vi "pH电极校准.vi"() -> ()   [LabVIEW 2016, in "斯坦道多参数.lvlib"]
uses:
  <vilib>/Utility/miscctls.llb/LVPointTypeDef.ctl
  <vilib>/Analysis/NI_AALBase.lvlib
panel:
  out "温度":dbl format="%#.2f"
  out "通讯状态":string
  out "电极状态标志":u16(ring) items=["OK", "第一点校正通过", "第二点校正通过", "校正失败,电极零点超出范围", "校正失败,电极斜率超出范围", "第三点校正通过"]
  in  "三点标液3":u16(ring)=6 caption="标液3" items=["TECH4.00", "TECH7.00", "TECH10.00", "NIST1.68", "NIST4.01", "NIST6.86", "NIST9.18", "NIST12.68"]
  in  "三点标液2":u16(ring)=5 caption="标液2" items=["TECH4.00", "TECH7.00", "TECH10.00", "NIST1.68", "NIST4.01", "NIST6.86", "NIST9.18", "NIST12.68"]
  in  "三点标液1":u16(ring)=4 caption="标液1" items=["TECH4.00", "TECH7.00", "TECH10.00", "NIST1.68", "NIST4.01", "NIST6.86", "NIST9.18", "NIST12.68"]
  out "第三点校准值":dbl
  in  "校准停止":bool
  in  "校准启动":bool
  out "第二点校准值":dbl
  out "第一点校准值":dbl
  out "提示":string
  in  "校准模式":enum16{"两点校准", "单点校准", "三点校准"}(ring)
  out "最小值":sgl format="%#.2f"
  out "最大值":sgl format="%#.2f"
  out "变异系数":dbl format="%#.6f"
  out "standard deviation":dbl caption="标准差" format="%#.2f"
  out "mean":dbl caption="均值" format="%#.2f"
  out "波形图表":sgl(graph) caption="历史曲线"
  out "当前检测值":dbl caption="测量值" format="%#.2f"
  out "标液2":dbl
  out "标液1":dbl
  out "当前信号值":dbl caption="信号值" format="%#.2f"
  out "偏移值补偿":dbl format="%#.2f"
  out "电极斜率":dbl format="%#.6f"
  out "电极零点":dbl format="%#.6f"
  # "酸碱度电极设定"
  # "℃"
  # "mV"
  # "mV"
  # "%"
  # "pH"
  # "请选择校准模式:"
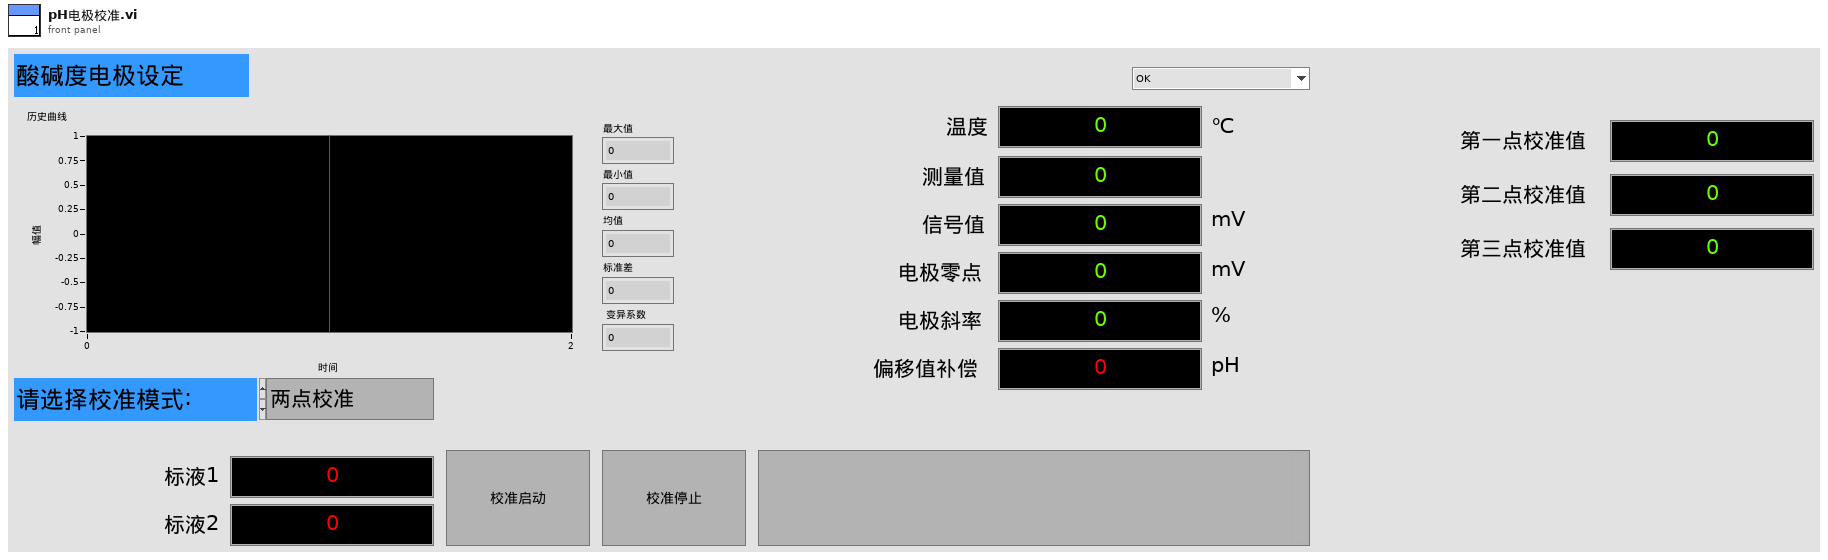
[diagram p1: front panel]
types:
  T1 = typedef "LVPointTypeDef.ctl" = cluster{"Horizontal":i16, "Vertical":i16}
  T2 = typedef "斯坦道多参数.lvlib/校准步骤.ctl" = enum16{"待机", "放置第一点标液", "第一点校准启动", "第一点校准写入", "第一点校准失败", "放置第二点标液", "第二点校准启动", "第二点校准写入", "第二点校准失败", "放置第三点标液", "第三点校准启动", "第三点校准写入", "第三点校准失败", "校准结果写入", "校准结束"}
  T3 = cluster{"电极状态标志":u16, "电极型号标志":u16, "酸碱度测量值":sgl, "温度测量值":sgl, "酸碱度信号值":sgl, "温度信号值":sgl, "酸碱度偏移修正值":sgl, "温度偏移修正值":sgl, "手动温度补偿值":sgl, "酸碱度电极零点":sgl, "酸碱度电极斜率":sgl, "第1点标准值记录":sgl, "第1点信号值记录":sgl, "第1点温度值记录":sgl, "第2点标准值记录":sgl, "第2点信号值记录":sgl, "第2点温度值记录":sgl, "命令滤波设定":u16, "温度模式":enum16{"ATC", "MTC"}, "生产批次":u16, "电极序号":u16, "串口地址":u16, "串口波特率":enum16{"9600", "19200", "115200"}, "串口校验位":enum16{"NONE", "ODD", "EVEN"}, "串口停止位":enum16{"1bit", "2bit"}, "第一点标准值":sgl, "第二点标准值":sgl}
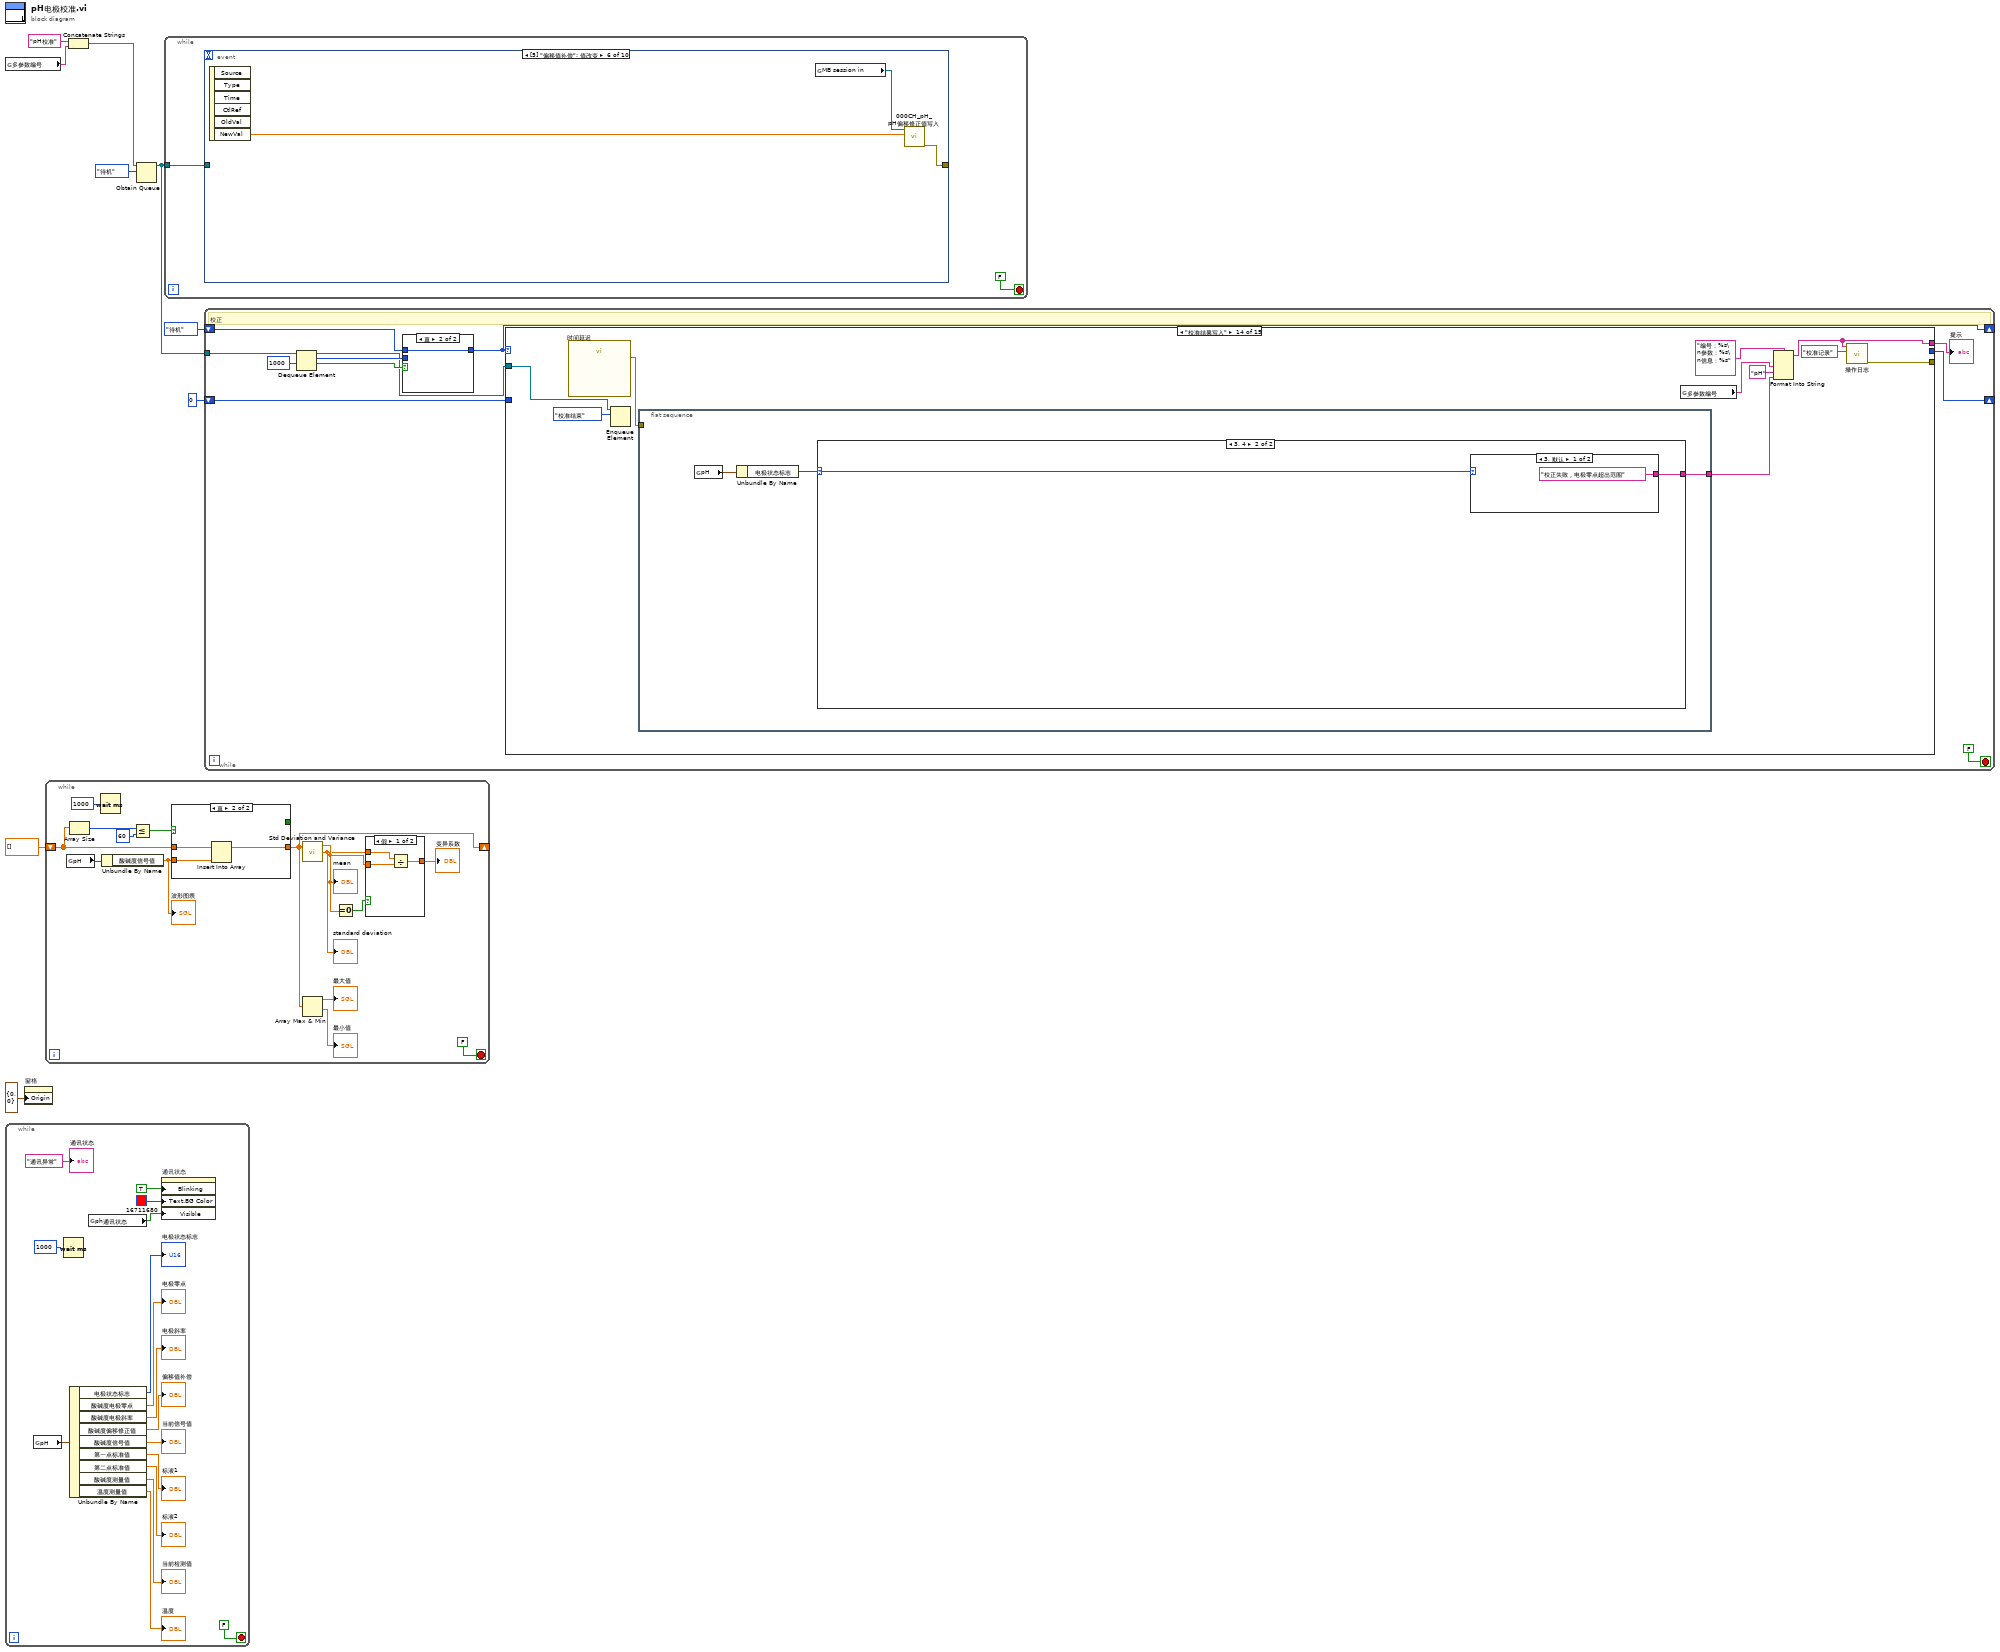
[diagram p0: block diagram]
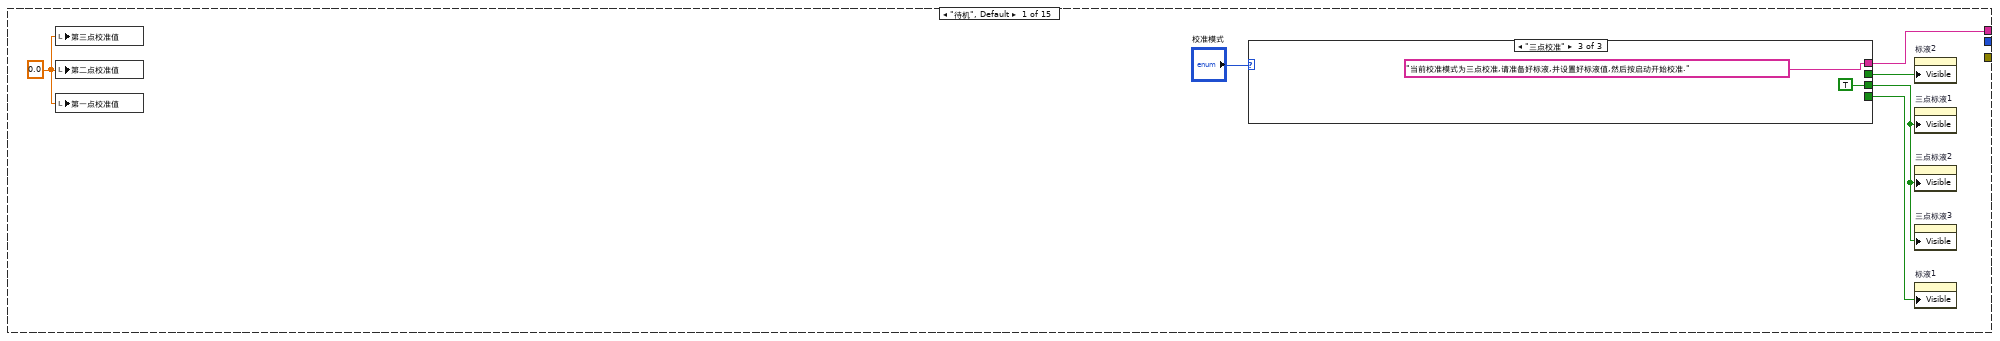
[diagram p3: hidden frame]
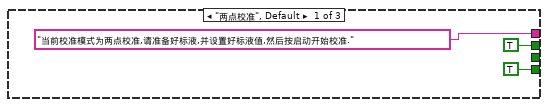
[diagram p4: hidden frame]
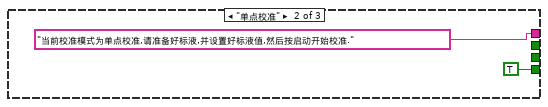
[diagram p5: hidden frame]
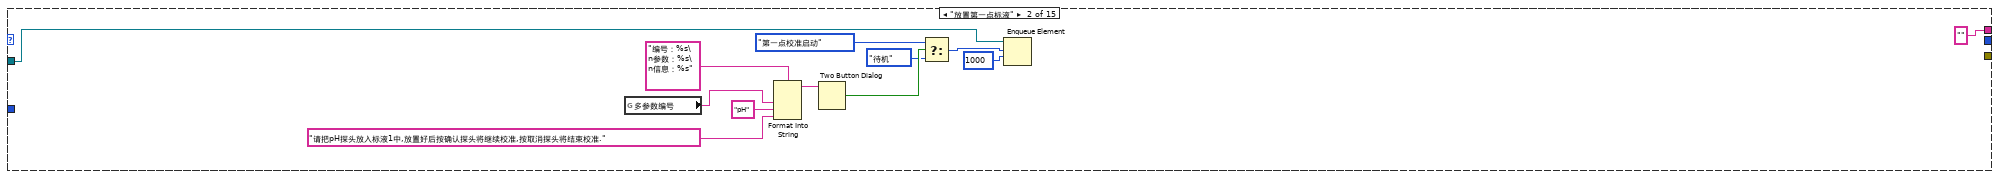
[diagram p6: hidden frame]
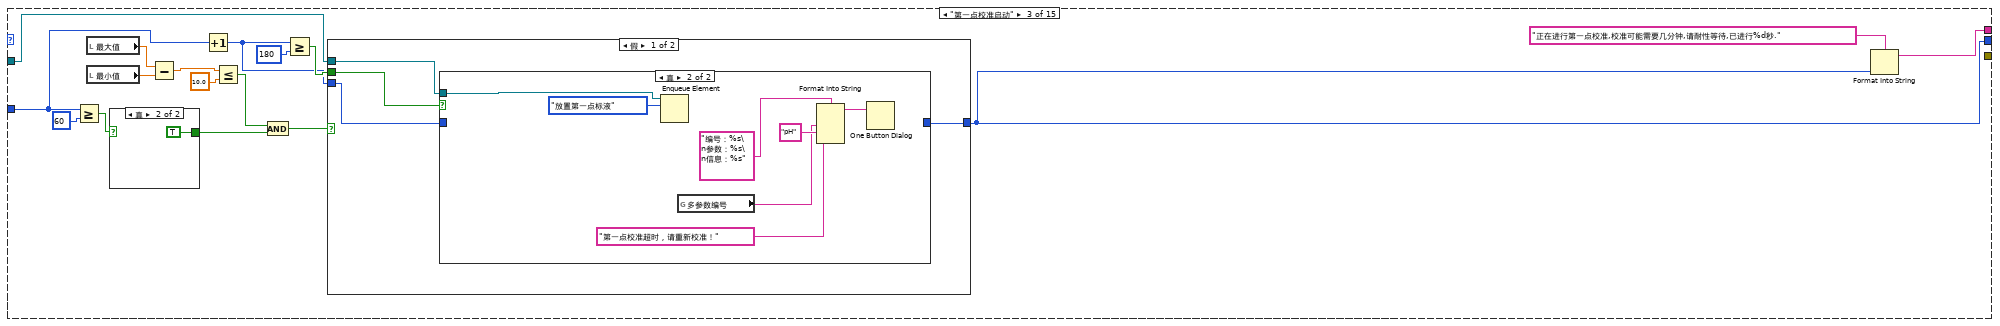
[diagram p7: hidden frame]
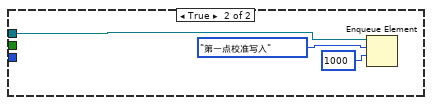
[diagram p9: hidden frame]
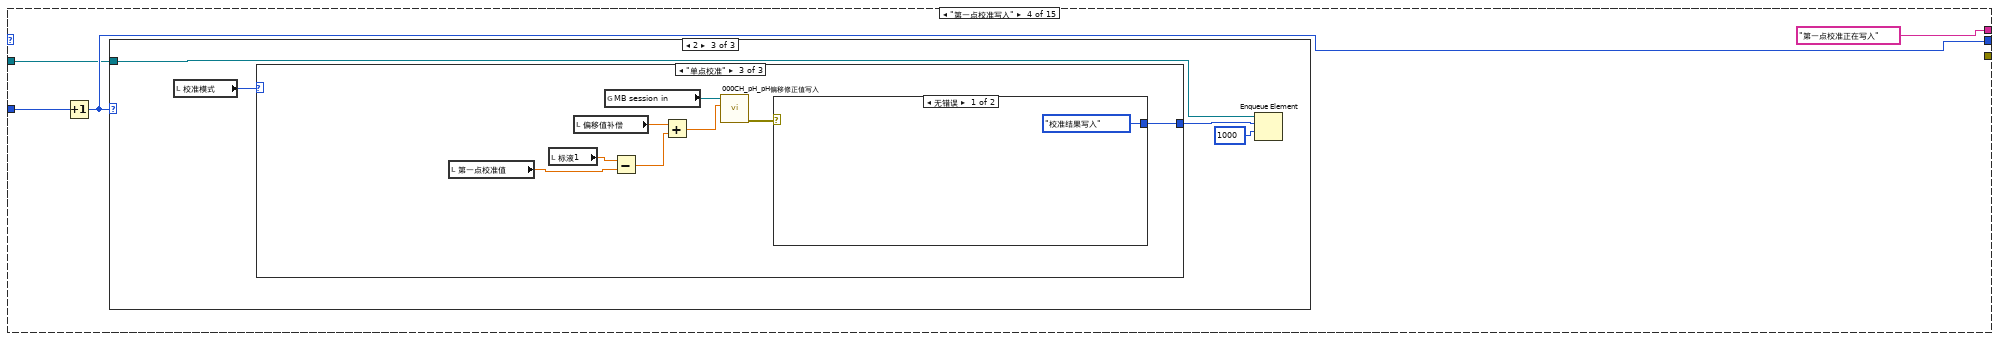
[diagram p11: hidden frame]
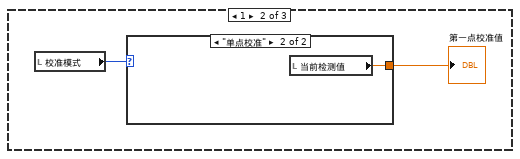
[diagram p13: hidden frame]
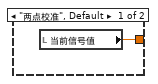
[diagram p14: hidden frame]
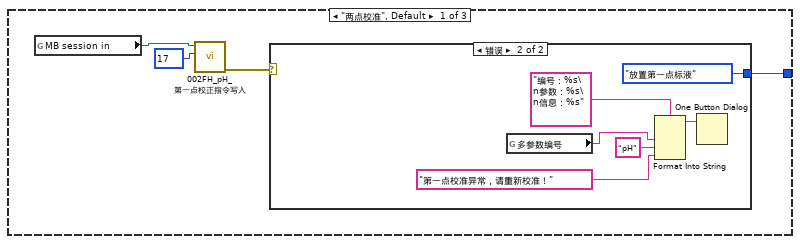
[diagram p15: hidden frame]
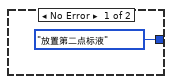
[diagram p16: hidden frame]
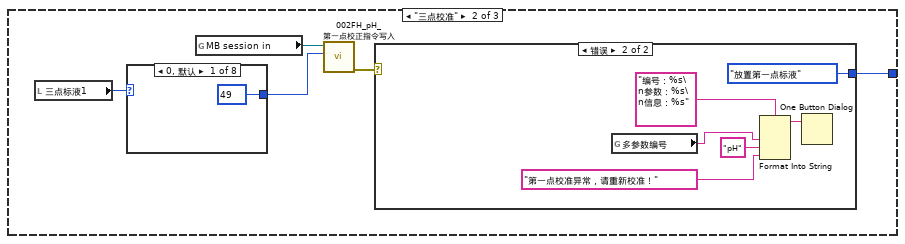
[diagram p17: hidden frame]
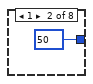
[diagram p18: hidden frame]
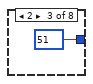
[diagram p19: hidden frame]
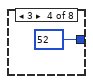
[diagram p20: hidden frame]
diagram:
  n1 = global read "多参数全局变量.vi" "多参数编号"() -> (w1:string)
  n2 = while {
    stop <- FALSE stop-if-true
    n3 = global read "国弘过程全局变量.vi" "pH"() -> (w23:T3)
    n4 = Wait (ms)(milliseconds to wait=u32 1000 ("等待时间（毫秒）")) -> ()  [unwired: 1 out]
    n5 = Unbundle By Name(w23) -> ("电极状态标志"=→"电极状态标志":u16, "酸碱度电极零点"=→"电极零点":sgl, "酸碱度电极斜率"=→"电极斜率":sgl, "酸碱度偏移修正值"=→"偏移值补偿":sgl, "酸碱度信号值"=→"当前信号值":sgl, "第一点标准值"=→"标液1":sgl, "第二点标准值"=→"标液2":sgl, "酸碱度测量值"=→"当前检测值":sgl, "温度测量值"=→"温度":sgl)
    n6 = global read "多参数全局变量.vi" "ph通讯状态"() -> (w12:bool)
    n7 = property on="通讯状态" class="Str"("Blinking"=TRUE ("闪烁"), "Text.BG Color"=u32 16711680, "Visible"=w12) -> ()  [unwired: 2 in, 2 out]
    "通讯状态" <- "通讯异常" ("当前串口")
  }
  n8 = property on="窗格" class="Pane"("Origin"=T1 {"Horizontal"=0, "Vertical"=0} ("原点")) -> ()  [unwired: 2 in, 2 out]
  n9 = while {
    shift-right: [w32] -> _
    shift-left: sgl[] [] -> [w36]
    stop <- FALSE stop-if-true
    n10 = global read "国弘过程全局变量.vi" "pH"() -> (w33:T3)
    n11 = Array Size(array=w36) -> (size(s)=w38:i32)
    n12 = Wait (ms)(milliseconds to wait=u32 1000 ("等待时间（毫秒）")) -> ()  [unwired: 1 out]
    n13 = Unbundle By Name(w33) -> ("酸碱度信号值"=w26:sgl)
    "波形图表" <- w26
    n14 = Less Or Equal?(x=w38, y=60) -> (x <= y?=w37:bool)
    n15 = case shown="真" w37 {
      tunnel: w36 -> [w49 w52]
      tunnel: w26 -> [w47 w51]
      tunnel: [w45 w50] -> w32
      tunnel: [TRUE _] -> _
      frame False {
        n16 = Replace Array Subset(array=w49, new element=w47) -> (w48:sgl[])  [unwired: 1 in]
        n17 = Rotate 1D Array(1:w48, 2:-1 ("n")) -> (0:w45:sgl[])
      }
      frame True {
        n18 = Insert Into Array(array=w52, new element=w51) -> (w50:sgl[])  [unwired: 1 in]
      }
    }
    n19 = call <vilib>:"Std Deviation and Variance.vi"("X"=w32) -> ("mean"=w28:dbl, "standard deviation"=w27:dbl)  [unwired: 1 in, 1 out]
    "mean" <- w28
    "standard deviation" <- w27
    n20 = Array Max & Min(array=w32) -> (max value=→"最大值":sgl, min value=→"最小值":sgl)  [unwired: 2 out]
    n21 = Equal To 0?(x=w28) -> (x = 0?=w35:bool)
    n22 = case shown="假" w35 {
      tunnel: w27 -> [w43 _]
      tunnel: [w42 _] -> w29
      tunnel: w28 -> [w41 _]
      frame False {
        n23 = Divide(x=w43, y=w41) -> (x/y=w42:dbl)
      }
      frame True {
      }
    }
    "变异系数" <- w29
  }
  n24 = Concatenate Strings("pH校准" ("名称（未命名）"), w1) -> (w2:string)
  n25 = Obtain Queue(name (unnamed)=w2, element data type=校准步骤."待机" ("枚举")) -> (queue out=w4:refnum<queue>)  [unwired: 3 in, 2 out]
  n26 = while {
    tunnel: w4 -> [w53]
    stop <- FALSE stop-if-true
    n27 = event shown="[5] \"偏移值补偿\": 值改变" {
      selector: _ -> [_ _ _ _ _ _ _ _ _ _]
      dyn-events: _ -> [_ _ _ _ _ _ _ _ _ _]
      timeout: _ -> [_ _ _ _ _ _ _ _ _ _]
      tunnel: [_ _ _ _ _ w105 w108 w111 _ _] -> _
      tunnel: w53 -> [_ _ _ _ _ _ _ _ w113 w115]
      event Timeout {
        n28 = event-data() -> ()  [unwired: 1 in, 3 out]
      }
      event "三点标液1": Value Change {
        n29 = event-data() -> ("NewVal"=w55:u16)  [unwired: 1 in, 5 out]
        n30 = case shown="0, 默认" w55 {
          frame 0, Default {
            w56 = u16 0 items=["TECH4.00", "TECH7.00", "TECH10.00", "NIST1.68", "NIST4.01", "NIST6.86", "NIST9.18", "NIST12.68"] ("标液2")
            w57 = u16 2 items=["TECH4.00", "TECH7.00", "TECH10.00", "NIST1.68", "NIST4.01", "NIST6.86", "NIST9.18", "NIST12.68"] ("标液3")
            w58 = u16 1 items=["TECH4.00", "TECH7.00", "TECH10.00", "NIST1.68", "NIST4.01", "NIST6.86", "NIST9.18", "NIST12.68"] ("标液2")
            n31 = local write "三点标液3"(w57) -> ()
            n32 = local write "三点标液2"(w58) -> ()
            n33 = local write "三点标液1"(w56) -> ()
          }
          frame 1 {
            w59 = u16 0 items=["TECH4.00", "TECH7.00", "TECH10.00", "NIST1.68", "NIST4.01", "NIST6.86", "NIST9.18", "NIST12.68"] ("标液2")
            w60 = u16 2 items=["TECH4.00", "TECH7.00", "TECH10.00", "NIST1.68", "NIST4.01", "NIST6.86", "NIST9.18", "NIST12.68"] ("标液3")
            w61 = u16 1 items=["TECH4.00", "TECH7.00", "TECH10.00", "NIST1.68", "NIST4.01", "NIST6.86", "NIST9.18", "NIST12.68"] ("标液2")
            n34 = local write "三点标液3"(w60) -> ()
            n35 = local write "三点标液2"(w61) -> ()
            n36 = local write "三点标液1"(w59) -> ()
          }
          frame 2 {
            w62 = u16 2 items=["TECH4.00", "TECH7.00", "TECH10.00", "NIST1.68", "NIST4.01", "NIST6.86", "NIST9.18", "NIST12.68"] ("标液2")
            w63 = u16 0 items=["TECH4.00", "TECH7.00", "TECH10.00", "NIST1.68", "NIST4.01", "NIST6.86", "NIST9.18", "NIST12.68"] ("标液3")
            w64 = u16 1 items=["TECH4.00", "TECH7.00", "TECH10.00", "NIST1.68", "NIST4.01", "NIST6.86", "NIST9.18", "NIST12.68"] ("标液2")
            n37 = local write "三点标液3"(w63) -> ()
            n38 = local write "三点标液2"(w64) -> ()
            n39 = local write "三点标液1"(w62) -> ()
          }
          frame 3 {
            w65 = u16 3 items=["TECH4.00", "TECH7.00", "TECH10.00", "NIST1.68", "NIST4.01", "NIST6.86", "NIST9.18", "NIST12.68"] ("标液2")
            w66 = u16 5 items=["TECH4.00", "TECH7.00", "TECH10.00", "NIST1.68", "NIST4.01", "NIST6.86", "NIST9.18", "NIST12.68"] ("标液3")
            w67 = u16 4 items=["TECH4.00", "TECH7.00", "TECH10.00", "NIST1.68", "NIST4.01", "NIST6.86", "NIST9.18", "NIST12.68"] ("标液2")
            n40 = local write "三点标液3"(w66) -> ()
            n41 = local write "三点标液2"(w67) -> ()
            n42 = local write "三点标液1"(w65) -> ()
          }
          frame 4 {
            w68 = u16 4 items=["TECH4.00", "TECH7.00", "TECH10.00", "NIST1.68", "NIST4.01", "NIST6.86", "NIST9.18", "NIST12.68"] ("标液2")
            w69 = u16 6 items=["TECH4.00", "TECH7.00", "TECH10.00", "NIST1.68", "NIST4.01", "NIST6.86", "NIST9.18", "NIST12.68"] ("标液3")
            w70 = u16 5 items=["TECH4.00", "TECH7.00", "TECH10.00", "NIST1.68", "NIST4.01", "NIST6.86", "NIST9.18", "NIST12.68"] ("标液2")
            n43 = local write "三点标液3"(w69) -> ()
            n44 = local write "三点标液2"(w70) -> ()
            n45 = local write "三点标液1"(w68) -> ()
          }
          frame 5..7 {
            w71 = u16 5 items=["TECH4.00", "TECH7.00", "TECH10.00", "NIST1.68", "NIST4.01", "NIST6.86", "NIST9.18", "NIST12.68"] ("标液2")
            w72 = u16 7 items=["TECH4.00", "TECH7.00", "TECH10.00", "NIST1.68", "NIST4.01", "NIST6.86", "NIST9.18", "NIST12.68"] ("标液3")
            w73 = u16 6 items=["TECH4.00", "TECH7.00", "TECH10.00", "NIST1.68", "NIST4.01", "NIST6.86", "NIST9.18", "NIST12.68"] ("标液2")
            n46 = local write "三点标液3"(w72) -> ()
            n47 = local write "三点标液2"(w73) -> ()
            n48 = local write "三点标液1"(w71) -> ()
          }
        }
      }
      event "三点标液2": Value Change {
        n49 = event-data() -> ("NewVal"=w74:u16)  [unwired: 1 in, 5 out]
        n50 = case shown="6, 7" w74 {
          frame 0..2, Default {
            w75 = u16 0 items=["TECH4.00", "TECH7.00", "TECH10.00", "NIST1.68", "NIST4.01", "NIST6.86", "NIST9.18", "NIST12.68"] ("标液2")
            w76 = u16 2 items=["TECH4.00", "TECH7.00", "TECH10.00", "NIST1.68", "NIST4.01", "NIST6.86", "NIST9.18", "NIST12.68"] ("标液3")
            w77 = u16 1 items=["TECH4.00", "TECH7.00", "TECH10.00", "NIST1.68", "NIST4.01", "NIST6.86", "NIST9.18", "NIST12.68"] ("标液2")
            n51 = local write "三点标液3"(w76) -> ()
            n52 = local write "三点标液2"(w77) -> ()
            n53 = local write "三点标液1"(w75) -> ()
          }
          frame 3, 4 {
            w78 = u16 3 items=["TECH4.00", "TECH7.00", "TECH10.00", "NIST1.68", "NIST4.01", "NIST6.86", "NIST9.18", "NIST12.68"] ("标液2")
            w79 = u16 5 items=["TECH4.00", "TECH7.00", "TECH10.00", "NIST1.68", "NIST4.01", "NIST6.86", "NIST9.18", "NIST12.68"] ("标液3")
            w80 = u16 4 items=["TECH4.00", "TECH7.00", "TECH10.00", "NIST1.68", "NIST4.01", "NIST6.86", "NIST9.18", "NIST12.68"] ("标液2")
            n54 = local write "三点标液3"(w79) -> ()
            n55 = local write "三点标液2"(w80) -> ()
            n56 = local write "三点标液1"(w78) -> ()
          }
          frame 5 {
            w81 = u16 6 items=["TECH4.00", "TECH7.00", "TECH10.00", "NIST1.68", "NIST4.01", "NIST6.86", "NIST9.18", "NIST12.68"] ("标液3")
            w82 = u16 5 items=["TECH4.00", "TECH7.00", "TECH10.00", "NIST1.68", "NIST4.01", "NIST6.86", "NIST9.18", "NIST12.68"] ("标液2")
            n57 = local write "三点标液3"(w81) -> ()
            n58 = local write "三点标液2"(w82) -> ()
          }
          frame 6, 7 {
            w83 = u16 7 items=["TECH4.00", "TECH7.00", "TECH10.00", "NIST1.68", "NIST4.01", "NIST6.86", "NIST9.18", "NIST12.68"] ("标液3")
            w84 = u16 6 items=["TECH4.00", "TECH7.00", "TECH10.00", "NIST1.68", "NIST4.01", "NIST6.86", "NIST9.18", "NIST12.68"] ("标液2")
            n59 = local write "三点标液3"(w83) -> ()
            n60 = local write "三点标液2"(w84) -> ()
          }
        }
      }
      event "三点标液3": Value Change {
        n61 = event-data() -> ("NewVal"=w85:u16)  [unwired: 1 in, 5 out]
        n62 = case shown="3..7" w85 {
          frame 0, 1, Default {
            w86 = u16 2 items=["TECH4.00", "TECH7.00", "TECH10.00", "NIST1.68", "NIST4.01", "NIST6.86", "NIST9.18", "NIST12.68"] ("标液2")
            w87 = u16 0 items=["TECH4.00", "TECH7.00", "TECH10.00", "NIST1.68", "NIST4.01", "NIST6.86", "NIST9.18", "NIST12.68"] ("标液3")
            w88 = u16 1 items=["TECH4.00", "TECH7.00", "TECH10.00", "NIST1.68", "NIST4.01", "NIST6.86", "NIST9.18", "NIST12.68"] ("标液2")
            n63 = local write "三点标液3"(w87) -> ()
            n64 = local write "三点标液2"(w88) -> ()
            n65 = local write "三点标液1"(w86) -> ()
          }
          frame 2 {
            w89 = u16 0 items=["TECH4.00", "TECH7.00", "TECH10.00", "NIST1.68", "NIST4.01", "NIST6.86", "NIST9.18", "NIST12.68"] ("标液2")
            w90 = u16 2 items=["TECH4.00", "TECH7.00", "TECH10.00", "NIST1.68", "NIST4.01", "NIST6.86", "NIST9.18", "NIST12.68"] ("标液3")
            w91 = u16 1 items=["TECH4.00", "TECH7.00", "TECH10.00", "NIST1.68", "NIST4.01", "NIST6.86", "NIST9.18", "NIST12.68"] ("标液2")
            n66 = local write "三点标液3"(w90) -> ()
            n67 = local write "三点标液2"(w91) -> ()
            n68 = local write "三点标液1"(w89) -> ()
          }
          frame 3..7 {
            n69 = local read "三点标液1"() -> (w94:u16)
            n70 = local read "三点标液2"() -> (w93:u16)
            n71 = Less?(x=w94, y=w93) -> (x < y?=w92:bool)
            n72 = case shown="假" w92 {
              frame False {
              }
              frame True {
                n73 = local read "三点标液3"() -> (w97:u16)
                n74 = local read "三点标液2"() -> (w95:u16)
                n75 = Less Or Equal?(x=w97, y=w95) -> (x <= y?=w96:bool)
                n76 = case shown="真" w96 {
                  tunnel: w95 -> [_ w99]
                  frame False {
                  }
                  frame True {
                    n77 = Increment(x=w99) -> (x+1=w98:u16)
                    n78 = local write "三点标液3"(w98) -> ()
                  }
                }
              }
            }
          }
        }
      }
      event "标液1", "标液2", "偏移值补偿": Mouse Down {
        n79 = event-data() -> ("CtlRef"=w103:refnum<vi>)  [unwired: 1 in, 7 out]
        n80 = property class="DigNum (严格)"(reference=w103) -> (reference out=w100:refnum<vi>, "Value"=w101:dbl)  [unwired: 1 in, 1 out]
        n81 = call "数字键盘.vi"("OldNumber"=w101) -> ("NewNumber"=w102:dbl)  [unwired: 1 in]
        n82 = property class="DigNum (严格)"(reference=w100, "Val(Sgnl)"=w102) -> ()  [unwired: 1 in, 2 out]
      }
      event "偏移值补偿": Value Change {
        n83 = event-data() -> ("NewVal"=w106:dbl)  [unwired: 1 in, 5 out]
        n84 = global read "多参数全局变量.vi" "MB session in"() -> (w104:refnum<class "MB_Master.lvclass">)
        n85 = call "000CH_pH_pH偏移修正值写入.vi"("数值"=w106, "MB session in"=w104) -> ("error out"=w105:errorcluster)  [unwired: 8 in, 1 out]
      }
      event "标液1": Value Change {
        n86 = event-data() -> ("NewVal"=w109:dbl)  [unwired: 1 in, 5 out]
        n87 = global read "多参数全局变量.vi" "MB session in"() -> (w107:refnum<class "MB_Master.lvclass">)
        n88 = call "0030H_pH_第一点标准值写入.vi"("数值"=w109, "MB session in"=w107) -> ("error out"=w108:errorcluster)  [unwired: 8 in, 1 out]
      }
      event "标液2": Value Change {
        n89 = event-data() -> ("NewVal"=w112:dbl)  [unwired: 1 in, 5 out]
        n90 = global read "多参数全局变量.vi" "MB session in"() -> (w110:refnum<class "MB_Master.lvclass">)
        n91 = call "0033H_pH_第二点标准值写入.vi"("数值"=w112, "MB session in"=w110) -> ("error out"=w111:errorcluster)  [unwired: 8 in, 1 out]
      }
      event "校准启动": Value Change {
        n92 = event-data() -> ()  [unwired: 1 in, 6 out]
        n93 = Enqueue Element(queue=w113, element=校准步骤."放置第一点标液" ("元素")) -> ()  [unwired: 2 in, 3 out]
      }
      event "校准停止": Value Change {
        n94 = event-data() -> ()  [unwired: 1 in, 6 out]
        n95 = Flush Queue(queue=w115) -> (queue out=w116:refnum<queue>)  [unwired: 1 in, 2 out]
        n96 = Enqueue Element(queue=w116, element=校准步骤."待机" ("元素"), timeout in ms (-1)=1000 ("超时毫秒(-1)")) -> ()  [unwired: 1 in, 3 out]
      }
    }
  }
  n97 = while "While循环" {
    shift-right: [w120] -> _
    shift-left: 校准步骤."待机" ("枚举") -> [w121]
    shift-right: [w127] -> _
    shift-left: 0 -> [w128]
    tunnel: w4 -> [w125]
    stop <- FALSE stop-if-true
    # "校正"
    n98 = Dequeue Element(queue=w125, timeout in ms (-1)=1000 ("超时毫秒(-1)")) -> (queue out=w119:refnum<queue>, element=w122:T2, timed out?=w123:bool)  [unwired: 1 in, 1 out]
    n99 = case shown="真" w123 {
      tunnel: w122 -> [w130 _]
      tunnel: [w130 w131] -> w120
      tunnel: w121 -> [_ w131]
      frame False {
      }
      frame True {
      }
    }
    n100 = case shown="\"校准结果写入\"" w120 {
      tunnel: [w137 "" ("提示") w172 "第一点校准正在写入" ("提示") _ "" ("提示") w275 "第二点校准正在写入" ("提示") _ "" ("提示") w360 "第三点校准正在写入" ("提示") _ w408 w442] -> w126
      tunnel: w128 -> [_ _ w166 w192 _ _ w269 w295 _ _ w354 w380 _ _ _]
      tunnel: [_ _ w157 w191 _ _ w260 w294 _ _ w345 w379 _ _ _] -> w127
      tunnel: w119 -> [_ w156 w160 w190 _ w259 w263 w293 _ w344 w348 w378 _ w414 _]
      tunnel: [_ _ _ _ _ _ _ _ _ _ _ _ _ w412 _] -> _
      frame "待机", Default {
        w133 = 0.0 ("第一点校准值")
        n101 = local write "第三点校准值"(w133) -> ()
        n102 = local write "第二点校准值"(w133) -> ()
        n103 = local write "第一点校准值"(w133) -> ()
        n104 = case shown="\"三点校准\"" "校准模式" {
          tunnel: ["当前校准模式为两点校准,请准备好标液,并设置好标液值,然后按启动开始校准." ("提示") "当前校准模式为单点校准,请准备好标液,并设置好标液值,然后按启动开始校准." ("提示") "当前校准模式为三点校准,请准备好标液,并设置好标液值,然后按启动开始校准." ("提示")] -> w137
          tunnel: [TRUE ("可见") _ _] -> w136
          tunnel: [TRUE ("可见") TRUE ("可见") _] -> w134
          tunnel: [_ _ TRUE ("可见")] -> w132
          frame "两点校准", Default {
          }
          frame "单点校准" {
          }
          frame "三点校准" {
          }
        }
        n105 = property on="标液2" class="DigNum (严格)"("Visible"=w136) -> ()  [unwired: 2 in, 2 out]
        n106 = property on="三点标液1" class="Ring (严格)"("Visible"=w132) -> ()  [unwired: 2 in, 2 out]
        n107 = property on="三点标液2" class="Ring (严格)"("Visible"=w132) -> ()  [unwired: 2 in, 2 out]
        n108 = property on="三点标液3" class="Ring (严格)"("Visible"=w132) -> ()  [unwired: 2 in, 2 out]
        n109 = property on="标液1" class="DigNum (严格)"("Visible"=w134) -> ()  [unwired: 2 in, 2 out]
      }
      frame "放置第一点标液" {
        n110 = global read "多参数全局变量.vi" "多参数编号"() -> (w148:string)
        n111 = Format Into String(format string="编号：%s\n参数：%s\n信息：%s" ("格式字符串"), w148, "pH" ("输入 2"), "请把pH探头放入标液1中,放置好后按确认探头将继续校准,按取消探头将结束校准." ("消息")) -> (resulting string=w145:string)  [unwired: 2 in, 1 out]
        n112 = Two Button Dialog(message=w145) -> (T button?=w154:bool)  [unwired: 2 in]
        n113 = Select(t=校准步骤."第一点校准启动" ("元素"), s=w154, f=校准步骤."待机" ("元素")) -> (s? t:f=w151:T2)
        n114 = Enqueue Element(queue=w156, element=w151, timeout in ms (-1)=1000 ("超时毫秒(-1)")) -> ()  [unwired: 1 in, 3 out]
      }
      frame "第一点校准启动" {
        n115 = Greater Or Equal?(x=w166, y=60) -> (x >= y?=w167:bool)
        n116 = local read "最大值"() -> (w163:sgl)
        n117 = local read "最小值"() -> (w164:sgl)
        n118 = case shown="真" w167 {
          tunnel: [_ TRUE] -> w165
          frame False {
          }
          frame True {
          }
        }
        n119 = Subtract(x=w163, y=w164) -> (x-y=w162:sgl)
        n120 = Increment(x=w166) -> (x+1=w158:i32)
        n121 = Less Or Equal?(x=w162, y=10.0) -> (x <= y?=w170:bool)
        n122 = And(x=w170, y=w165) -> (x .and. y?=w161:bool)
        n123 = Greater Or Equal?(x=w158, y=180) -> (x >= y?=w159:bool)
        n124 = case shown="假" w161 {
          tunnel: w160 -> [w176 w188]
          tunnel: w159 -> [w177 _]
          tunnel: w158 -> [w175 _]
          tunnel: [w174 _] -> w157
          frame False {
            n125 = case shown="真" w177 {
              tunnel: w176 -> [_ w185]
              tunnel: w175 -> [w178 _]
              tunnel: [w178 _] -> w174
              frame False {
              }
              frame True {
                n126 = Enqueue Element(queue=w185, element=校准步骤."放置第一点标液" ("元素")) -> ()  [unwired: 2 in, 3 out]
                n127 = global read "多参数全局变量.vi" "多参数编号"() -> (w180:string)
                n128 = Format Into String(format string="编号：%s\n参数：%s\n信息：%s" ("格式字符串"), w180, "pH" ("输入 2"), "第一点校准超时，请重新校准！" ("error source (\" \")")) -> (resulting string=w182:string)  [unwired: 2 in, 1 out]
                n129 = One Button Dialog(message=w182) -> ()  [unwired: 1 in, 1 out]
              }
            }
          }
          frame True {
            n130 = Enqueue Element(queue=w188, element=校准步骤."第一点校准写入" ("元素"), timeout in ms (-1)=1000 ("超时毫秒(-1)")) -> ()  [unwired: 1 in, 3 out]
          }
        }
        n131 = Format Into String(format string="正在进行第一点校准,校准可能需要几分钟,请耐性等待,已进行%d秒." ("格式字符串"), w157) -> (resulting string=w172:string)  [unwired: 2 in, 1 out]
      }
      frame "第一点校准写入" {
        n132 = Increment(x=w192) -> (x+1=w191:i32)
        n133 = case shown="2" w191 {
          tunnel: w190 -> [_ _ w201]
          frame 0, Default {
          }
          frame 1 {
            n134 = local read "校准模式"() -> (w194:enum16{"两点校准", "单点校准", "三点校准"})
            n135 = case shown="\"单点校准\"" w194 {
              tunnel: [w196 w197] -> w195
              frame "两点校准", Default {
                n136 = local read "当前信号值"() -> (w196:dbl)
              }
              frame "单点校准" {
                n137 = local read "当前检测值"() -> (w197:dbl)
              }
            }
            "第一点校准值" <- w195
          }
          frame 2 {
            n138 = local read "校准模式"() -> (w200:enum16{"两点校准", "单点校准", "三点校准"})
            n139 = case shown="\"单点校准\"" w200 {
              tunnel: [w205 w217 w235] -> w199
              frame "两点校准", Default {
                n140 = global read "多参数全局变量.vi" "MB session in"() -> (w204:refnum<class "MB_Master.lvclass">)
                n141 = call "002FH_pH_第一点校正指令写入.vi"("数值"=u16 17, "MB session in"=w204) -> ("error out"=w202:errorcluster)  [unwired: 8 in, 1 out]
                n142 = case shown="错误" w202 {
                  tunnel: [校准步骤."放置第二点标液" ("元素") 校准步骤."放置第一点标液" ("元素")] -> w205
                  frame No Error {
                  }
                  frame Error {
                    n143 = global read "多参数全局变量.vi" "多参数编号"() -> (w208:string)
                    n144 = Format Into String(format string="编号：%s\n参数：%s\n信息：%s" ("格式字符串"), w208, "pH" ("输入 2"), "第一点校准异常，请重新校准！" ("error source (\" \")")) -> (resulting string=w210:string)  [unwired: 2 in, 1 out]
                    n145 = One Button Dialog(message=w210) -> ()  [unwired: 1 in, 1 out]
                  }
                }
              }
              frame "三点校准" {
                n146 = local read "三点标液1"() -> (w214:u16)
                n147 = case shown="0, 默认" w214 {
                  tunnel: [u16 49 ("数值") u16 50 ("数值") u16 51 ("数值") u16 52 ("数值") u16 53 ("数值") u16 54 ("数值") u16 55 ("数值") u16 56 ("数值")] -> w213
                  frame 0, Default {
                  }
                  frame 1 {
                  }
                  frame 2 {
                  }
                  frame 3 {
                  }
                  frame 4 {
                  }
                  frame 5 {
                  }
                  frame 6 {
                  }
                  frame 7 {
                  }
                }
                n148 = global read "多参数全局变量.vi" "MB session in"() -> (w216:refnum<class "MB_Master.lvclass">)
                n149 = call "002FH_pH_第一点校正指令写入.vi"("数值"=w213, "MB session in"=w216) -> ("error out"=w215:errorcluster)  [unwired: 8 in, 1 out]
                n150 = case shown="错误" w215 {
                  tunnel: [校准步骤."放置第二点标液" ("元素") 校准步骤."放置第一点标液" ("元素")] -> w217
                  frame No Error {
                  }
                  frame Error {
                    n151 = global read "多参数全局变量.vi" "多参数编号"() -> (w228:string)
                    n152 = Format Into String(format string="编号：%s\n参数：%s\n信息：%s" ("格式字符串"), w228, "pH" ("输入 2"), "第一点校准异常，请重新校准！" ("error source (\" \")")) -> (resulting string=w230:string)  [unwired: 2 in, 1 out]
                    n153 = One Button Dialog(message=w230) -> ()  [unwired: 1 in, 1 out]
                  }
                }
              }
              frame "单点校准" {
                n154 = local read "第一点校准值"() -> (w240:dbl)
                n155 = local read "标液1"() -> (w239:dbl)
                n156 = local read "偏移值补偿"() -> (w233:dbl)
                n157 = global read "多参数全局变量.vi" "MB session in"() -> (w238:refnum<class "MB_Master.lvclass">)
                n158 = Subtract(x=w239, y=w240) -> (x-y=w237:dbl)
                n159 = Add(x=w233, y=w237) -> (x+y=w234:dbl)
                n160 = call "000CH_pH_pH偏移修正值写入.vi"("数值"=w234, "MB session in"=w238) -> ("error out"=w236:errorcluster)  [unwired: 8 in, 1 out]
                n161 = case shown="无错误" w236 {
                  tunnel: [校准步骤."校准结果写入" ("元素") 校准步骤."放置第一点标液" ("元素")] -> w235
                  frame No Error {
                  }
                  frame Error {
                    n162 = global read "多参数全局变量.vi" "多参数编号"() -> (w245:string)
                    n163 = Format Into String(format string="编号：%s\n参数：%s\n信息：%s" ("格式字符串"), w245, "pH" ("输入 2"), "校准异常，请重新校准！" ("error source (\" \")")) -> (resulting string=w243:string)  [unwired: 2 in, 1 out]
                    n164 = One Button Dialog(message=w243) -> ()  [unwired: 1 in, 1 out]
                  }
                }
              }
            }
            n165 = Enqueue Element(queue=w201, element=w199, timeout in ms (-1)=1000 ("超时毫秒(-1)")) -> ()  [unwired: 1 in, 3 out]
          }
        }
      }
      frame "第一点校准失败" {
      }
      frame "放置第二点标液" {
        n166 = global read "多参数全局变量.vi" "多参数编号"() -> (w251:string)
        n167 = Format Into String(format string="编号：%s\n参数：%s\n信息：%s" ("格式字符串"), w251, "pH" ("输入 2"), "请把探头放入标液2中,放置好后按确认探头将继续校准,按取消探头将结束校准." ("消息")) -> (resulting string=w248:string)  [unwired: 2 in, 1 out]
        n168 = Two Button Dialog(message=w248) -> (T button?=w257:bool)  [unwired: 2 in]
        n169 = Select(t=校准步骤."第二点校准启动" ("元素"), s=w257, f=校准步骤."待机" ("元素")) -> (s? t:f=w254:T2)
        n170 = Enqueue Element(queue=w259, element=w254, timeout in ms (-1)=1000 ("超时毫秒(-1)")) -> ()  [unwired: 1 in, 3 out]
      }
      frame "第二点校准启动" {
        n171 = Greater Or Equal?(x=w269, y=60) -> (x >= y?=w270:bool)
        n172 = local read "最大值"() -> (w266:sgl)
        n173 = local read "最小值"() -> (w267:sgl)
        n174 = case shown="真" w270 {
          tunnel: [_ TRUE] -> w268
          frame False {
          }
          frame True {
          }
        }
        n175 = Subtract(x=w266, y=w267) -> (x-y=w265:sgl)
        n176 = Increment(x=w269) -> (x+1=w261:i32)
        n177 = Less Or Equal?(x=w265, y=10.0) -> (x <= y?=w273:bool)
        n178 = And(x=w273, y=w268) -> (x .and. y?=w264:bool)
        n179 = Greater Or Equal?(x=w261, y=180) -> (x >= y?=w262:bool)
        n180 = case shown="假" w264 {
          tunnel: w263 -> [w279 w291]
          tunnel: w262 -> [w280 _]
          tunnel: w261 -> [w278 _]
          tunnel: [w277 _] -> w260
          frame False {
            n181 = case shown="真" w280 {
              tunnel: w279 -> [_ w288]
              tunnel: w278 -> [w281 _]
              tunnel: [w281 _] -> w277
              frame False {
              }
              frame True {
                n182 = Enqueue Element(queue=w288, element=校准步骤."放置第二点标液" ("元素")) -> ()  [unwired: 2 in, 3 out]
                n183 = global read "多参数全局变量.vi" "多参数编号"() -> (w283:string)
                n184 = Format Into String(format string="编号：%s\n参数：%s\n信息：%s" ("格式字符串"), w283, "pH" ("输入 2"), "第二点校准超时，请重新校准！" ("error source (\" \")")) -> (resulting string=w285:string)  [unwired: 2 in, 1 out]
                n185 = One Button Dialog(message=w285) -> ()  [unwired: 1 in, 1 out]
              }
            }
          }
          frame True {
            n186 = Enqueue Element(queue=w291, element=校准步骤."第二点校准写入" ("元素"), timeout in ms (-1)=1000 ("超时毫秒(-1)")) -> ()  [unwired: 1 in, 3 out]
          }
        }
        n187 = Format Into String(format string="正在进行第二点校准,校准可能需要几分钟,请耐性等待,已进行%d秒." ("格式字符串"), w260) -> (resulting string=w275:string)  [unwired: 2 in, 1 out]
      }
      frame "第二点校准写入" {
        n188 = Increment(x=w295) -> (x+1=w294:i32)
        n189 = case shown="1" w294 {
          tunnel: w293 -> [_ _ w301]
          frame 0, Default {
          }
          frame 1 {
            n190 = local read "当前信号值"() -> (→"第二点校准值":dbl)
          }
          frame 2 {
            n191 = local read "校准模式"() -> (w298:enum16{"两点校准", "单点校准", "三点校准"})
            n192 = case shown="\"三点校准\"" w298 {
              tunnel: [w302 w315] -> w299
              frame "两点校准", Default {
                n193 = global read "多参数全局变量.vi" "MB session in"() -> (w304:refnum<class "MB_Master.lvclass">)
                n194 = call "0032H_pH_第二点校正指令写入.vi"("数值"=u16 33, "MB session in"=w304) -> ("error out"=w303:errorcluster)  [unwired: 8 in, 1 out]
                n195 = case shown="错误" w303 {
                  tunnel: [校准步骤."校准结果写入" ("元素") 校准步骤."放置第二点标液" ("元素")] -> w302
                  frame No Error {
                  }
                  frame Error {
                    n196 = global read "多参数全局变量.vi" "多参数编号"() -> (w308:string)
                    n197 = Format Into String(format string="编号：%s\n参数：%s\n信息：%s" ("格式字符串"), w308, "pH" ("输入 2"), "第二点校准异常，请重新校准！" ("error source (\" \")")) -> (resulting string=w310:string)  [unwired: 2 in, 1 out]
                    n198 = One Button Dialog(message=w310) -> ()  [unwired: 1 in, 1 out]
                  }
                }
              }
              frame "三点校准" {
                n199 = local read "三点标液2"() -> (w314:u16)
                n200 = case shown="7" w314 {
                  tunnel: [u16 49 ("数值") u16 50 ("数值") u16 51 ("数值") u16 52 ("数值") u16 53 ("数值") u16 54 ("数值") u16 55 ("数值") u16 56 ("数值")] -> w313
                  frame 0, Default {
                  }
                  frame 1 {
                  }
                  frame 2 {
                  }
                  frame 3 {
                  }
                  frame 4 {
                  }
                  frame 5 {
                  }
                  frame 6 {
                  }
                  frame 7 {
                  }
                }
                n201 = global read "多参数全局变量.vi" "MB session in"() -> (w317:refnum<class "MB_Master.lvclass">)
                n202 = call "0032H_pH_第二点校正指令写入.vi"("数值"=w313, "MB session in"=w317) -> ("error out"=w316:errorcluster)  [unwired: 8 in, 1 out]
                n203 = case shown="错误" w316 {
                  tunnel: [校准步骤."放置第三点标液" ("元素") 校准步骤."放置第二点标液" ("元素")] -> w315
                  frame No Error {
                  }
                  frame Error {
                    n204 = global read "多参数全局变量.vi" "多参数编号"() -> (w328:string)
                    n205 = Format Into String(format string="编号：%s\n参数：%s\n信息：%s" ("格式字符串"), w328, "pH" ("输入 2"), "第二点校准异常，请重新校准！" ("error source (\" \")")) -> (resulting string=w330:string)  [unwired: 2 in, 1 out]
                    n206 = One Button Dialog(message=w330) -> ()  [unwired: 1 in, 1 out]
                  }
                }
              }
            }
            n207 = Enqueue Element(queue=w301, element=w299, timeout in ms (-1)=1000 ("超时毫秒(-1)")) -> ()  [unwired: 1 in, 3 out]
          }
        }
      }
      frame "第二点校准失败" {
      }
      frame "放置第三点标液" {
        n208 = global read "多参数全局变量.vi" "多参数编号"() -> (w336:string)
        n209 = Format Into String(format string="编号：%s\n参数：%s\n信息：%s" ("格式字符串"), w336, "pH" ("输入 2"), "请把探头放入标液3中,放置好后按确认探头将继续校准,按取消探头将结束校准." ("消息")) -> (resulting string=w333:string)  [unwired: 2 in, 1 out]
        n210 = Two Button Dialog(message=w333) -> (T button?=w342:bool)  [unwired: 2 in]
        n211 = Select(t=校准步骤."第三点校准启动" ("元素"), s=w342, f=校准步骤."待机" ("元素")) -> (s? t:f=w339:T2)
        n212 = Enqueue Element(queue=w344, element=w339, timeout in ms (-1)=1000 ("超时毫秒(-1)")) -> ()  [unwired: 1 in, 3 out]
      }
      frame "第三点校准启动" {
        n213 = Greater Or Equal?(x=w354, y=60) -> (x >= y?=w355:bool)
        n214 = local read "最大值"() -> (w351:sgl)
        n215 = local read "最小值"() -> (w352:sgl)
        n216 = case shown="真" w355 {
          tunnel: [_ TRUE] -> w353
          frame False {
          }
          frame True {
          }
        }
        n217 = Subtract(x=w351, y=w352) -> (x-y=w350:sgl)
        n218 = Increment(x=w354) -> (x+1=w346:i32)
        n219 = Less Or Equal?(x=w350, y=10.0) -> (x <= y?=w358:bool)
        n220 = And(x=w358, y=w353) -> (x .and. y?=w349:bool)
        n221 = Greater Or Equal?(x=w346, y=180) -> (x >= y?=w347:bool)
        n222 = case shown="假" w349 {
          tunnel: w348 -> [w364 w376]
          tunnel: w347 -> [w365 _]
          tunnel: w346 -> [w363 _]
          tunnel: [w362 _] -> w345
          frame False {
            n223 = case shown="真" w365 {
              tunnel: w364 -> [_ w373]
              tunnel: w363 -> [w366 _]
              tunnel: [w366 _] -> w362
              frame False {
              }
              frame True {
                n224 = Enqueue Element(queue=w373, element=校准步骤."待机" ("元素")) -> ()  [unwired: 2 in, 3 out]
                n225 = global read "多参数全局变量.vi" "多参数编号"() -> (w368:string)
                n226 = Format Into String(format string="编号：%s\n参数：%s\n信息：%s" ("格式字符串"), w368, "pH" ("输入 2"), "第三点校准超时，请重新校准！" ("error source (\" \")")) -> (resulting string=w370:string)  [unwired: 2 in, 1 out]
                n227 = One Button Dialog(message=w370) -> ()  [unwired: 1 in, 1 out]
              }
            }
          }
          frame True {
            n228 = Enqueue Element(queue=w376, element=校准步骤."第三点校准写入" ("元素"), timeout in ms (-1)=1000 ("超时毫秒(-1)")) -> ()  [unwired: 1 in, 3 out]
          }
        }
        n229 = Format Into String(format string="正在进行第三点校准,校准可能需要几分钟,请耐性等待,已进行%d秒." ("格式字符串"), w345) -> (resulting string=w360:string)  [unwired: 2 in, 1 out]
      }
      frame "第三点校准写入" {
        n230 = Increment(x=w380) -> (x+1=w379:i32)
        n231 = case shown="1" w379 {
          tunnel: w378 -> [_ _ w389]
          frame 0, Default {
          }
          frame 1 {
            n232 = local read "当前信号值"() -> (→"第三点校准值":dbl)
          }
          frame 2 {
            n233 = local read "三点标液3"() -> (w384:u16)
            n234 = case shown="0, 默认" w384 {
              tunnel: [u16 49 ("数值") u16 50 ("数值") u16 51 ("数值") u16 52 ("数值") u16 53 ("数值") u16 54 ("数值") u16 55 ("数值") u16 56 ("数值")] -> w383
              frame 0, Default {
              }
              frame 1 {
              }
              frame 2 {
              }
              frame 3 {
              }
              frame 4 {
              }
              frame 5 {
              }
              frame 6 {
              }
              frame 7 {
              }
            }
            n235 = global read "多参数全局变量.vi" "MB session in"() -> (w386:refnum<class "MB_Master.lvclass">)
            n236 = call "0035H_pH_第三点校正指令写入.vi"("数值"=w383, "MB session in"=w386) -> ("error out"=w385:errorcluster)  [unwired: 8 in, 1 out]
            n237 = case shown="无错误" w385 {
              tunnel: [校准步骤."校准结果写入" ("元素") 校准步骤."第三点校准写入" ("元素")] -> w387
              frame No Error {
              }
              frame Error {
                n238 = global read "多参数全局变量.vi" "多参数编号"() -> (w400:string)
                n239 = Format Into String(format string="编号：%s\n参数：%s\n信息：%s" ("格式字符串"), w400, "pH" ("输入 2"), "第三点校准异常，请重新校准！" ("error source (\" \")")) -> (resulting string=w402:string)  [unwired: 2 in, 1 out]
                n240 = One Button Dialog(message=w402) -> ()  [unwired: 1 in, 1 out]
              }
            }
            n241 = Enqueue Element(queue=w389, element=w387, timeout in ms (-1)=1000 ("超时毫秒(-1)")) -> ()  [unwired: 1 in, 3 out]
          }
        }
      }
      frame "第三点校准失败" {
      }
      frame "校准结果写入" {
        n242 = call "时间延迟"() -> ("error out"=w406:errorcluster)  [unwired: 11 in]
        n243 = Enqueue Element(queue=w414, element=校准步骤."校准结束" ("元素")) -> ()  [unwired: 2 in, 3 out]
        n244 = flat-sequence {
          tunnel: [w417] -> w407
          tunnel: w406 -> [_]
          frame #0 {
            n245 = global read "国弘过程全局变量.vi" "pH"() -> (w416:T3)
            n246 = Unbundle By Name(w416) -> ("电极状态标志"=w415:u16)
            n247 = case shown="3, 4" w415 {
              selector: w415 -> [_ w439]
              tunnel: [w418 w438] -> w417
              frame 0, Default {
                n248 = local read "校准模式"() -> (w419:enum16{"两点校准", "单点校准", "三点校准"})
                n249 = case shown="\"两点校准\", 默认" w419 {
                  tunnel: [w425 w433 w437] -> w418
                  frame "两点校准", Default {
                    n250 = local read "第一点校准值"() -> (w423:dbl)
                    n251 = local read "第二点校准值"() -> (w421:dbl)
                    n252 = local read "标液1"() -> (w424:dbl)
                    n253 = local read "标液2"() -> (w420:dbl)
                    n254 = Format Into String(format string="校准结果：第一点校准值=%f mV，第一点标准值=%f,第二点校准值=%f mV，第二点标准值=%f." ("提示"), w423, w424, w421, w420) -> (resulting string=w425:string)  [unwired: 2 in, 1 out]
                  }
                  frame "三点校准" {
                    n255 = local read "第一点校准值"() -> (w432:dbl)
                    n256 = local read "第二点校准值"() -> (w431:dbl)
                    n257 = local read "第三点校准值"() -> (w429:dbl)
                    n258 = property on="三点标液1" class="Ring (严格)"() -> ("RingText.Text"=w428:string)  [unwired: 2 in, 2 out]
                    n259 = property on="三点标液2" class="Ring (严格)"() -> ("RingText.Text"=w426:string)  [unwired: 2 in, 2 out]
                    n260 = property on="三点标液3" class="Ring (严格)"() -> ("RingText.Text"=w427:string)  [unwired: 2 in, 2 out]
                    n261 = Format Into String(format string="校准结果：第一点校准值=%f mV，第一点标准值=%s,第二点校准值=%f mV，第二点标准值=%s,第三点校准值=%f mV，第三点标准值=%s." ("提示"), w432, w428, w431, w426, w429, w427) -> (resulting string=w433:string)  [unwired: 2 in, 1 out]
                  }
                  frame "单点校准" {
                    n262 = local read "第一点校准值"() -> (w436:dbl)
                    n263 = local read "标液1"() -> (w434:dbl)
                    n264 = Format Into String(format string="校准结果：校准值=%f，标准值=%f。" ("提示"), w436, w434) -> (resulting string=w437:string)  [unwired: 2 in, 1 out]
                  }
                }
              }
              frame 3, 4 {
                n265 = case shown="3, 默认" w439 {
                  tunnel: ["校正失败，电极零点超出范围" "校正失败，电极斜率超出范围"] -> w438
                  frame 3, Default {
                  }
                  frame 4 {
                  }
                }
              }
            }
          }
        }
        n266 = global read "多参数全局变量.vi" "多参数编号"() -> (w410:string)
        n267 = Format Into String(format string="编号：%s\n参数：%s\n信息：%s" ("格式字符串"), w410, "pH" ("输入 2"), w407) -> (resulting string=w408:string)  [unwired: 2 in, 1 out]
        n268 = call "操作日志.vi"("table"="校准记录", "日志信息"=w408) -> ("error out"=w412:errorcluster)  [unwired: 9 in]
      }
      frame "校准结束" {
        n269 = local read "提示"() -> (w442:string)
      }
    }
    "提示" <- w126
  }
